vi "Demo.vi"() -> ()   [LabVIEW 2010]
uses:
  LinkedList.ctl
  Node.ctl
panel:
  out "Array":string[](array[string])
  # "Does not work yet."
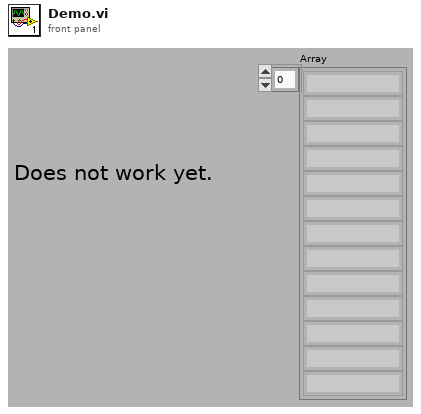
[diagram p1: front panel]
types:
  T1 = typedef "LinkedList.ctl" = cluster{"Root":refnum<data-value>, "Iterator":refnum<data-value>}
  T2 = typedef "Node.ctl" = cluster{"Name":string, "Next":variant, "Previous":variant}
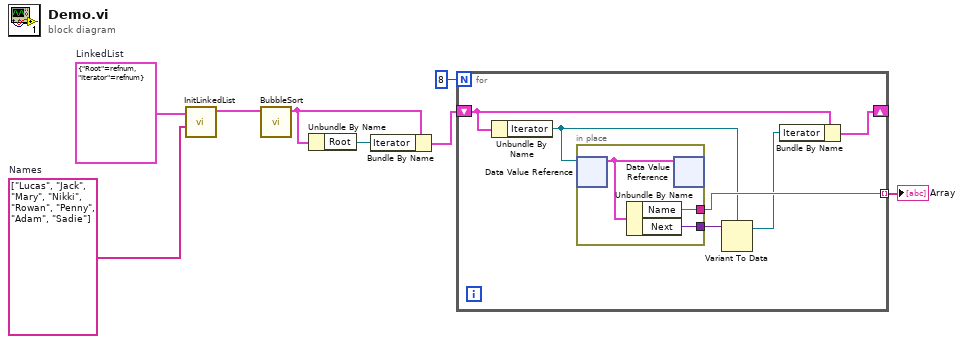
[diagram p0: block diagram]
diagram:
  w8 = T1 {"Root"=refnum, "Iterator"=refnum}  # LinkedList
  w7 = string[] ["Lucas", "Jack", "Mary", "Nikki", "Rowan", "Penny", "Adam", "Sadie"]  # Names
  n1 = call "InitLinkedList.vi"("Names"=w7, "LinkedList in"=w8) -> ("LinkedList out"=w6:T1)  [unwired: 9 in]
  n2 = call "BubbleSort.vi"("LinkedList in"=w6) -> ("LinkedList out"=w4:T1)  [unwired: 10 in]
  n3 = Unbundle By Name(w4) -> ("Root"=w3:refnum<data-value>)
  n4 = Bundle By Name(cluster=w4, "Iterator"=w3) -> (w2:T1)
  n5 = for {
    N: 8 -> [_]
    shift-right: [w9] -> _
    shift-left: w2 -> [w11]
    tunnel: [w14] -> w1 mode=indexing
    n6 = Unbundle By Name(w11) -> ("Iterator"=w12:refnum<data-value>)
    n7 = in-place {
      in-place-border: [w17] -> w14
      in-place-border: [w16] -> w13
      n8 = in-place-dvr #1(w12) -> (w15:T2)  [unwired: 1 out]
      n9 = Unbundle By Name(w15) -> ("Name"=w17:string, "Next"=w16:variant)
      n10 = in-place-dvr #1(w15) -> ()  [unwired: 2 out]
    }
    n11 = Variant To Data(Variant=w13, type=w12) -> (data=w10:refnum<data-value>)  [unwired: 1 in, 1 out]
    n12 = Bundle By Name(cluster=w11, "Iterator"=w10) -> (w9:T1)
  }
  "Array" <- w1
